vi "maincapactor.vi"() -> ()   [LabVIEW 2020]
panel:
  out "dup directory path":path
  in  "GPIB address magnet":string="1"
  in  "GPIB address Temp Controler":string="12"
  in  "GPIB address CapBridge":string="6"
  in  "Wait (minute)":u32
  in  "No of Temp Steps":i16
  in  "folder name to save files":string
  out "outputtemp":dbl[](array[numeric]) format="%.2f"
  out "outputdc":dbl[](array[numeric]) format="%.2f"
  out "outputcapacitor":dbl[](array[numeric]) format="%.2f"
  out "field":dbl[](array[numeric]) format="%.2f"
  out "Current Temp":dbl format="%.3f"
  in  "Increasing \nTemp step":bool=TRUE
  in  "Temperature\nInterval":dbl format="%.3f"
  in  "Initial Temp C":dbl format="%.3f"
  # "Help:\n1. write the folder name to save the files.The file name will \nbe the temperature in the given folder.\n2.Write the GPIB address of all the instruments before running\nthe program.\n3. Give the initial temperature and the temperature interval \nand the total number of steps.\n4.Check whether you want to increase the temperature or\ndecrease.\n5.Write the time to be waited to let the tempetature controller\nequilibrate.\n6.Once the speps 1 through 5 is done run the experiment."
  # "Decreasing\nTemp Step"
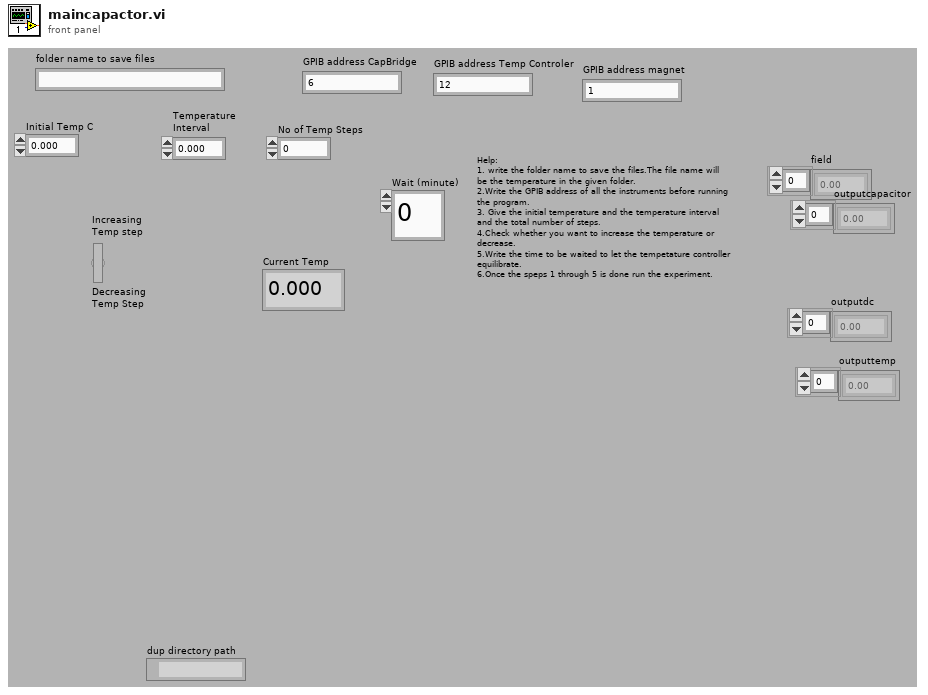
[diagram p1: front panel]
types:
  T1 = enum16{"--Quit--", "Read-Status", "Read-Cell", "Read-Field[T]", "Read-Setpoint[T]"}
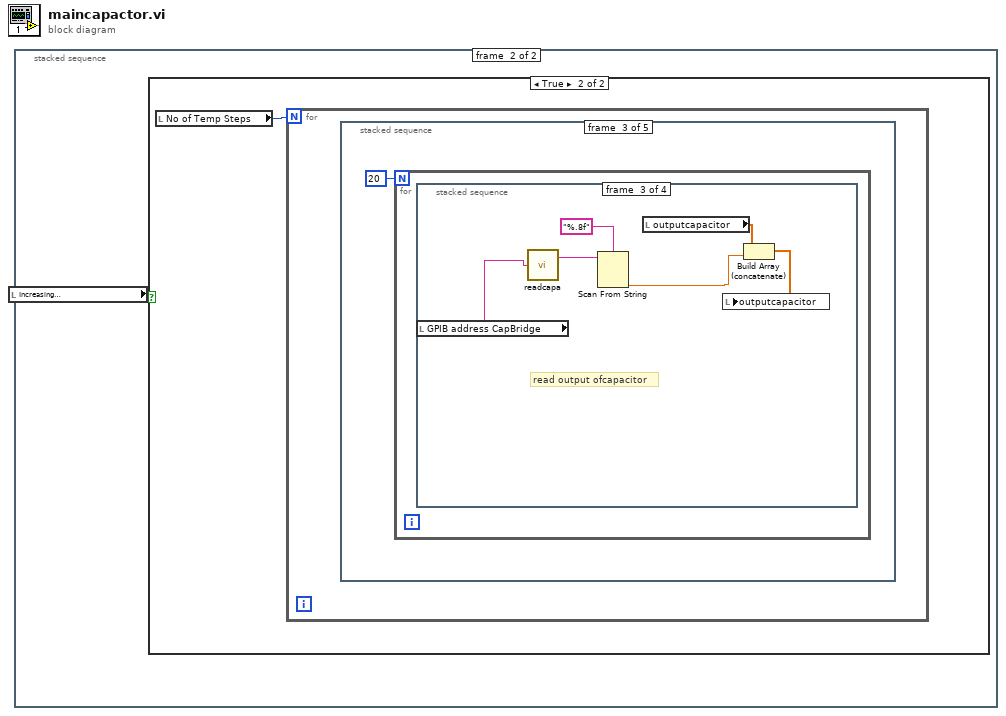
[diagram p0: block diagram]
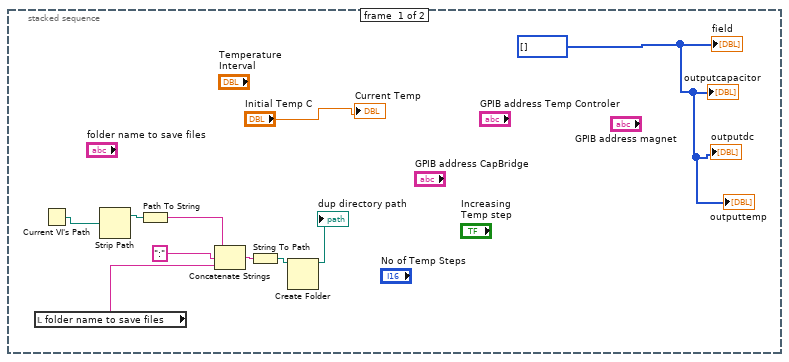
[diagram p2: hidden frame]
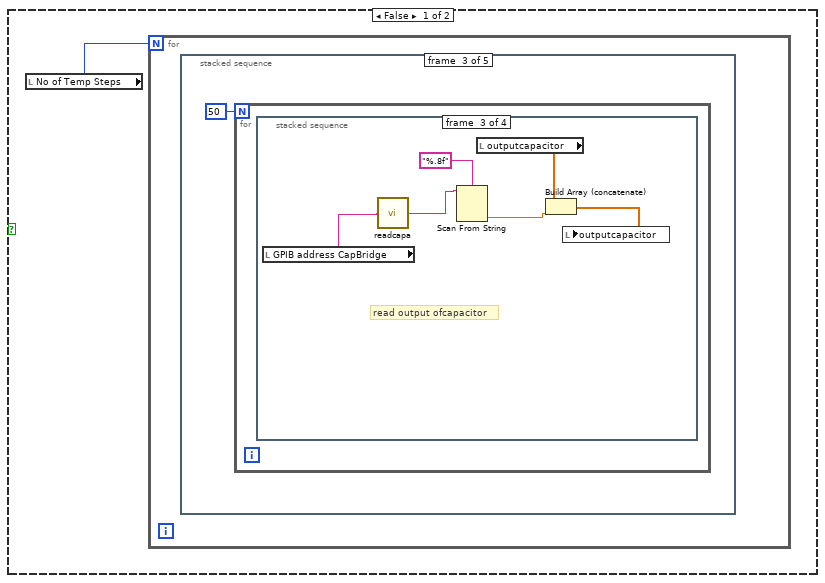
[diagram p3: hidden frame]
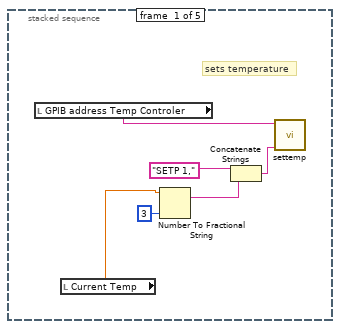
[diagram p4: hidden frame]
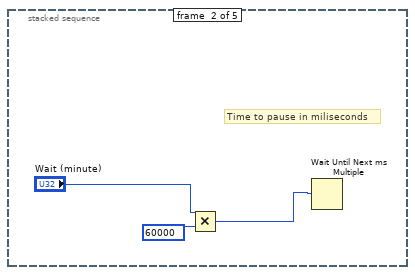
[diagram p5: hidden frame]
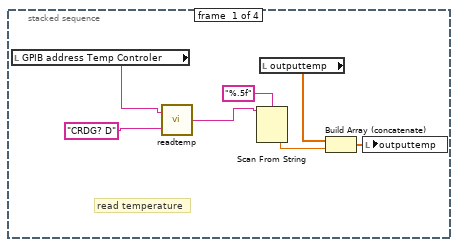
[diagram p6: hidden frame]
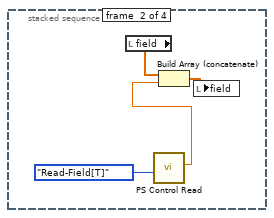
[diagram p7: hidden frame]
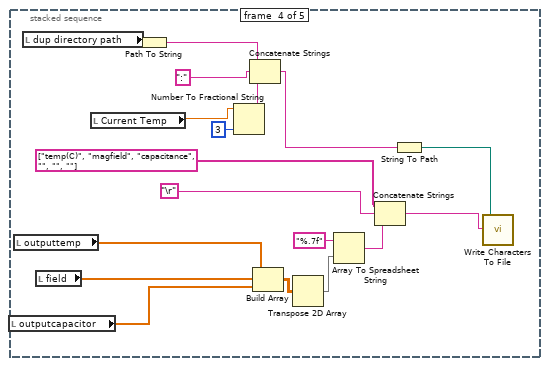
[diagram p9: hidden frame]
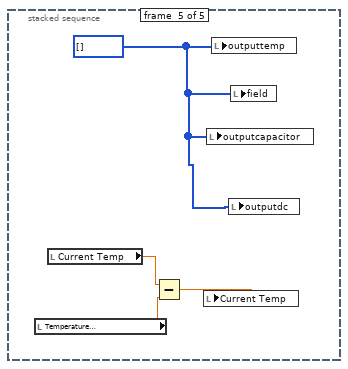
[diagram p10: hidden frame]
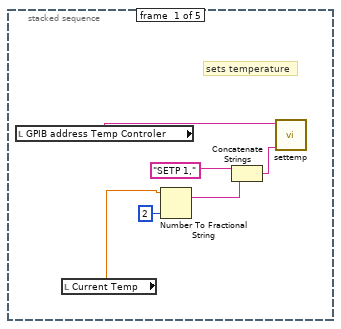
[diagram p11: hidden frame]
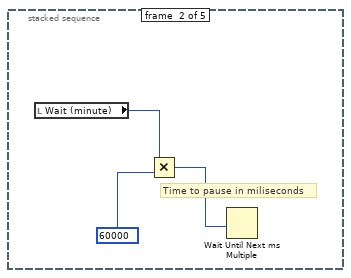
[diagram p12: hidden frame]
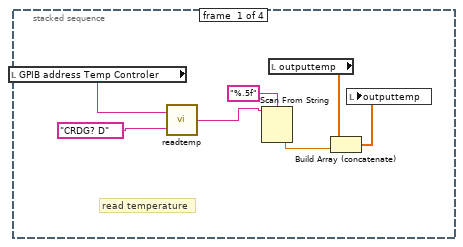
[diagram p13: hidden frame]
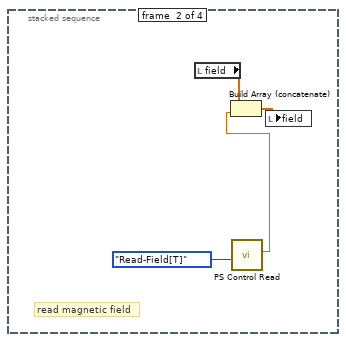
[diagram p14: hidden frame]
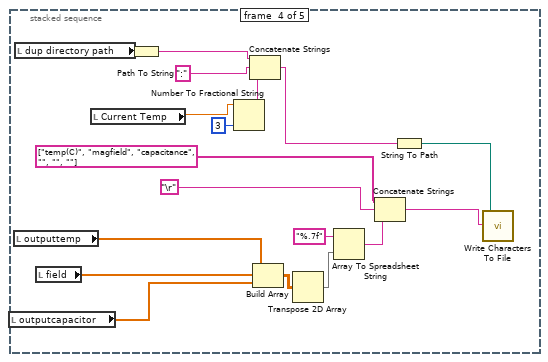
[diagram p16: hidden frame]
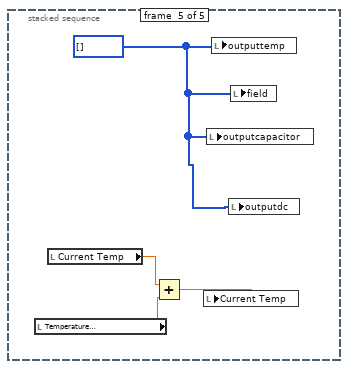
[diagram p17: hidden frame]
diagram:
  n1 = stacked-sequence {
    frame #0 {
      w9 = i32[] [] ("field")
      n2 = local read "folder name to save files"() -> (w4:string)
      n3 = Current VI's Path() -> (path=w8:path)
      n4 = Strip Path(path=w8) -> (stripped path=w7:path)  [unwired: 1 out]
      n5 = Path To String(path=w7) -> (string=w6:string)
      n6 = Concatenate Strings(w6, ":", w4) -> (w3:string)
      n7 = String To Path(string=w3) -> (path=w2:path)
      n8 = Create Folder(path (use dialog)=w2) -> (created path=→"dup directory path":path)  [unwired: 2 in, 2 out]
      "Current Temp" <- "Initial Temp C"
      "field" <- w9
      "outputcapacitor" <- w9
      "outputdc" <- w9
      "outputtemp" <- w9
    }
    frame #1 {
      n9 = local read "Increasing \nTemp step"() -> (w11:bool)
      n10 = case shown="True" w11 {
        frame False {
          n11 = local read "No of Temp Steps"() -> (w12:i16)
          n12 = for {
            N: w12 -> [_]
            n13 = stacked-sequence {
              frame #0 {
                # "sets temperature"
                n14 = local read "GPIB address Temp Controler"() -> (w13:string)
                n15 = local read "Current Temp"() -> (w15:dbl)
                n16 = Number To Fractional String(number=w15, precision (6)=i16 3) -> (F-format string=w18:string)  [unwired: 2 in]
                n17 = Concatenate Strings("SETP 1,", w18) -> (w16:string)
                n18 = call "settemp.vi"("Characters to Write"=w16, "GPIB\nAddress"=w13) -> ()  [unwired: 5 in, 1 out]
              }
              frame #1 {
                # "Time to pause in miliseconds"
                n19 = Multiply(x="Wait (minute)", y=60000) -> (x*y=w19:u32)
                n20 = Wait Until Next ms Multiple(millisecond multiple=w19) -> ()  [unwired: 1 out]
              }
              frame #2 {
                n21 = for {
                  N: 50 -> [_]
                  n22 = stacked-sequence {
                    frame #0 {
                      # "read temperature"
                      n23 = local read "GPIB address Temp Controler"() -> (w25:string)
                      n24 = call "readtemp.vi"("Characters to Write"="CRDG? D", "GPIB\nAddress"=w25) -> ("Characters Read"=w26:string)
                      n25 = Scan From String(format string="%.5f", input string=w26) -> (output 1=w23:dbl)  [unwired: 3 in, 3 out]
                      n26 = local read "outputtemp"() -> (w24:dbl[])
                      n27 = Build Array (concatenate)(w24, w23) -> (w29:dbl[])
                      n28 = local write "outputtemp"(w29) -> ()
                    }
                    frame #1 {
                      n29 = local read "field"() -> (w32:dbl[])
                      n30 = call "PS Control Read.vi"("Read State"=T1."Read-Field[T]") -> ("Current Field"=w30:dbl)  [unwired: 3 in, 4 out]
                      n31 = Build Array (concatenate)(w32, w30) -> (w33:dbl[])
                      n32 = local write "field"(w33) -> ()
                    }
                    frame #2 {
                      # "read output ofcapacitor"
                      n33 = local read "GPIB address CapBridge"() -> (w36:string)
                      n34 = call "readcapa.vi"("GPIB\nAddress"=w36) -> ("Characters Read"=w37:string)
                      n35 = Scan From String(format string="%.8f", input string=w37) -> (output 1=w34:dbl)  [unwired: 3 in, 3 out]
                      n36 = local read "outputcapacitor"() -> (w35:dbl[])
                      n37 = Build Array (concatenate)(w35, w34) -> (w39:dbl[])
                      n38 = local write "outputcapacitor"(w39) -> ()
                    }
                    frame #3 {
                      # "pause if needed"
                    }
                  }
                }
              }
              frame #3 {
                n39 = local read "outputcapacitor"() -> (w42:dbl[])
                n40 = local read "outputtemp"() -> (w52:dbl[])
                n41 = local read "dup directory path"() -> (w41:path)
                n42 = local read "field"() -> (w51:dbl[])
                n43 = local read "Current Temp"() -> (w54:dbl)
                n44 = Path To String(path=w41) -> (string=w40:string)
                n45 = Number To Fractional String(number=w54, precision (6)=i16 3) -> (F-format string=w53:string)  [unwired: 2 in]
                n46 = Concatenate Strings(w40, ":", w53) -> (w56:string)
                n47 = Build Array(w52, w51, w42) -> (w50:dbl[][])
                n48 = Transpose 2D Array(2D array=w50) -> (transposed array=w48:dbl[][])
                n49 = Array To Spreadsheet String(array=w48, 3:"%.7f" ("format string")) -> (spreadsheet string=w45:string)  [unwired: 1 in]
                n50 = Concatenate Strings(string[] ["temp(C)", "magfield", "capacitance", "", "", ""], "\r", w45) -> (w44:string)
                n51 = String To Path(string=w56) -> (path=w55:path)
                n52 = call <vilib>:"Write Characters To File.vi"("character string"=w44, "file path (dialog if empty)"=w55) -> ()  [unwired: 3 in, 1 out]
              }
              frame #4 {
                w61 = i32[] []
                n53 = local read "Temperature\nInterval"() -> (w59:dbl)
                n54 = local read "Current Temp"() -> (w60:dbl)
                n55 = Subtract(x=w60, y=w59) -> (x-y=w58:dbl)
                n56 = local write "Current Temp"(w58) -> ()
                n57 = local write "outputcapacitor"(w61) -> ()
                n58 = local write "outputtemp"(w61) -> ()
                n59 = local write "outputdc"(w61) -> ()
                n60 = local write "field"(w61) -> ()
              }
            }
          }
        }
        frame True {
          n61 = local read "No of Temp Steps"() -> (w62:i16)
          n62 = for {
            N: w62 -> [_]
            n63 = stacked-sequence {
              frame #0 {
                # "sets temperature"
                n64 = local read "GPIB address Temp Controler"() -> (w63:string)
                n65 = local read "Current Temp"() -> (w65:dbl)
                n66 = Number To Fractional String(number=w65, precision (6)=i16 2) -> (F-format string=w68:string)  [unwired: 2 in]
                n67 = Concatenate Strings("SETP 1,", w68) -> (w66:string)
                n68 = call "settemp.vi"("Characters to Write"=w66, "GPIB\nAddress"=w63) -> ()  [unwired: 5 in, 1 out]
              }
              frame #1 {
                # "Time to pause in miliseconds"
                n69 = local read "Wait (minute)"() -> (w71:u32)
                n70 = Multiply(x=w71, y=u32 60000 ("millisecond multiple")) -> (x*y=w69:u32)
                n71 = Wait Until Next ms Multiple(millisecond multiple=w69) -> ()  [unwired: 1 out]
              }
              frame #2 {
                n72 = for {
                  N: 20 -> [_]
                  n73 = stacked-sequence {
                    frame #0 {
                      # "read temperature"
                      n74 = local read "GPIB address Temp Controler"() -> (w75:string)
                      n75 = call "readtemp.vi"("Characters to Write"="CRDG? D", "GPIB\nAddress"=w75) -> ("Characters Read"=w76:string)
                      n76 = Scan From String(format string="%.5f", input string=w76) -> (output 1=w73:dbl)  [unwired: 3 in, 3 out]
                      n77 = local read "outputtemp"() -> (w74:dbl[])
                      n78 = Build Array (concatenate)(w74, w73) -> (w79:dbl[])
                      n79 = local write "outputtemp"(w79) -> ()
                    }
                    frame #1 {
                      # "read magnetic field"
                      n80 = local read "field"() -> (w82:dbl[])
                      n81 = call "PS Control Read.vi"("Read State"=T1."Read-Field[T]") -> ("Current Field"=w80:dbl)  [unwired: 3 in, 4 out]
                      n82 = Build Array (concatenate)(w82, w80) -> (w83:dbl[])
                      n83 = local write "field"(w83) -> ()
                    }
                    frame #2 {
                      # "read output ofcapacitor"
                      n84 = local read "GPIB address CapBridge"() -> (w86:string)
                      n85 = call "readcapa.vi"("GPIB\nAddress"=w86) -> ("Characters Read"=w87:string)
                      n86 = Scan From String(format string="%.8f", input string=w87) -> (output 1=w84:dbl)  [unwired: 3 in, 3 out]
                      n87 = local read "outputcapacitor"() -> (w85:dbl[])
                      n88 = Build Array (concatenate)(w85, w84) -> (w89:dbl[])
                      n89 = local write "outputcapacitor"(w89) -> ()
                    }
                    frame #3 {
                      # "pause if needed to take readings"
                    }
                  }
                }
              }
              frame #3 {
                n90 = local read "outputcapacitor"() -> (w92:dbl[])
                n91 = local read "outputtemp"() -> (w102:dbl[])
                n92 = local read "dup directory path"() -> (w91:path)
                n93 = local read "field"() -> (w101:dbl[])
                n94 = local read "Current Temp"() -> (w104:dbl)
                n95 = Path To String(path=w91) -> (string=w90:string)
                n96 = Number To Fractional String(number=w104, precision (6)=i16 3) -> (F-format string=w103:string)  [unwired: 2 in]
                n97 = Concatenate Strings(w90, ":", w103) -> (w106:string)
                n98 = Build Array(w102, w101, w92) -> (w100:dbl[][])
                n99 = Transpose 2D Array(2D array=w100) -> (transposed array=w98:dbl[][])
                n100 = Array To Spreadsheet String(array=w98, 3:"%.7f" ("format string")) -> (spreadsheet string=w95:string)  [unwired: 1 in]
                n101 = Concatenate Strings(string[] ["temp(C)", "magfield", "capacitance", "", "", ""], "\r", w95) -> (w94:string)
                n102 = String To Path(string=w106) -> (path=w105:path)
                n103 = call <vilib>:"Write Characters To File.vi"("character string"=w94, "file path (dialog if empty)"=w105) -> ()  [unwired: 3 in, 1 out]
              }
              frame #4 {
                w111 = i32[] []
                n104 = local read "Temperature\nInterval"() -> (w109:dbl)
                n105 = local read "Current Temp"() -> (w110:dbl)
                n106 = Add(x=w110, y=w109) -> (x+y=w108:dbl)
                n107 = local write "Current Temp"(w108) -> ()
                n108 = local write "outputcapacitor"(w111) -> ()
                n109 = local write "outputtemp"(w111) -> ()
                n110 = local write "outputdc"(w111) -> ()
                n111 = local write "field"(w111) -> ()
              }
            }
          }
        }
      }
    }
  }
